vi "Tarea 17.vi"() -> ()   [LabVIEW 2019]
uses:
  Student Material/Student Material/Module 4/Exercises 17/CLD 17 Keypad_Typedef.ctl
panel:
  out "error out":errorcluster
  in  "error in (no error)":errorcluster
  out "Numeric":dbl
  in  "Keypad Cluster":T1
  out "String":string="0"
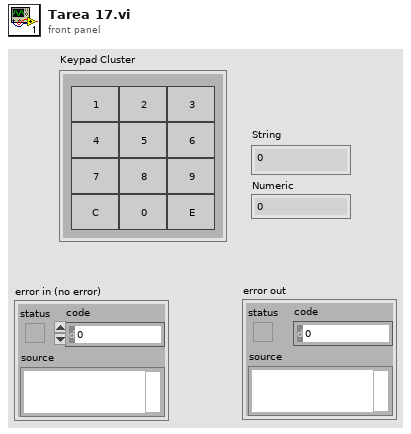
[diagram p1: front panel]
types:
  T1 = typedef "CLD 17 Keypad_Typedef.ctl" = cluster{"0":bool, "1":bool, "2":bool, "3":bool, "4":bool, "5":bool, "6":bool, "7":bool, "8":bool, "9":bool, "C":bool, "E":bool}
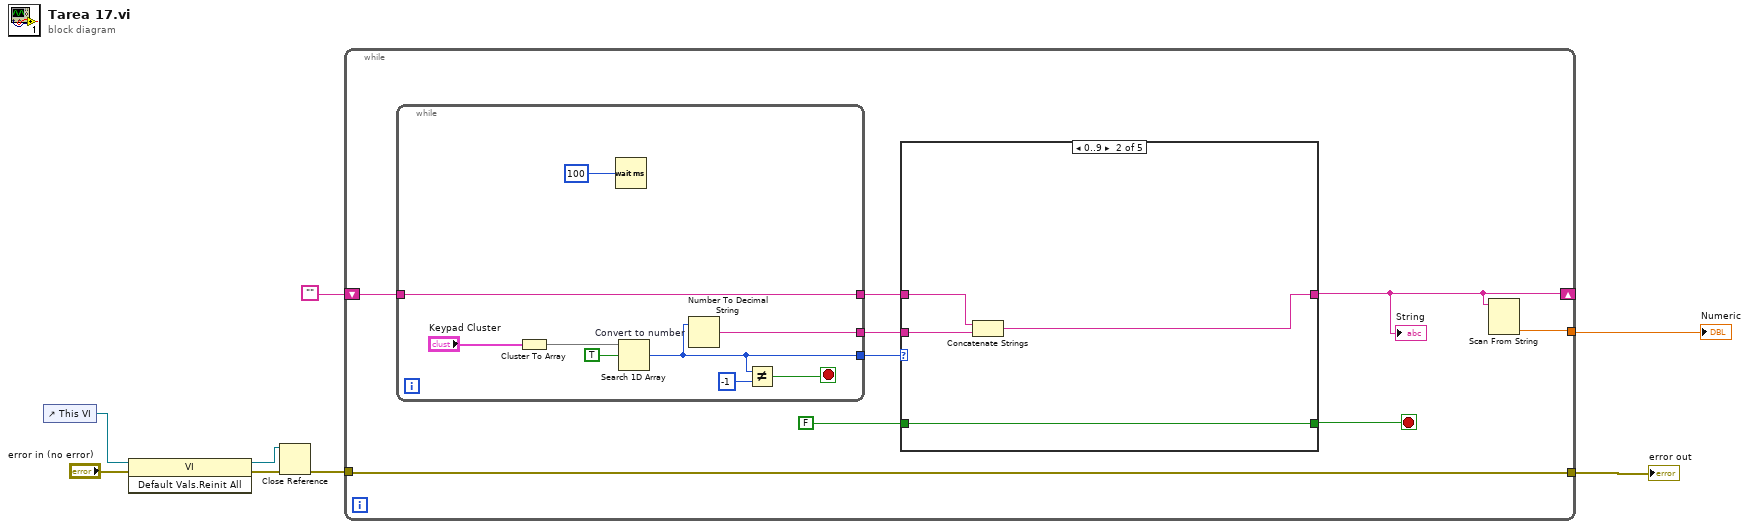
[diagram p0: block diagram]
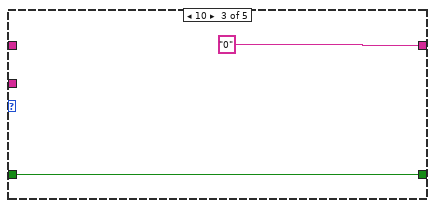
[diagram p3: hidden frame]
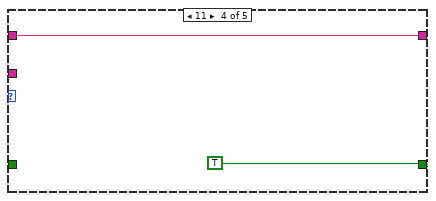
[diagram p4: hidden frame]
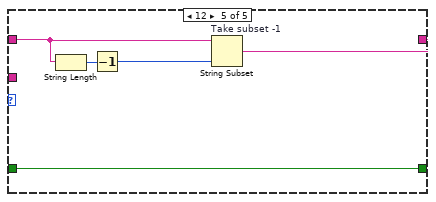
[diagram p5: hidden frame]
diagram:
  n1 = control-ref of="This VI"() -> (w7:refnum<vi>)
  n2 = invoke class="VI" method="Default Vals.Reinit All"(reference=w7, error in="error in (no error)") -> (reference out=w4:refnum<vi>, error out=w6:errorcluster)  [unwired: 1 in, 1 out]
  n3 = Close Reference(reference=w4, error in (no error)=w6) -> (error out=w5:errorcluster)
  n4 = while {
    shift-right: [w14] -> _
    shift-left: "" -> [w11]
    tunnel: w5 -> [w9]
    tunnel: [w17] -> w3
    tunnel: [w9] -> w1
    stop <- w13 stop-if-true
    n5 = while "Keypad Polling" {
      tunnel: [w34] -> w16
      tunnel: [w39] -> w15
      tunnel: [w38] -> w10
      tunnel: w11 -> [w38]
      stop <- w35 stop-if-true
      n6 = Cluster To Array(cluster="Keypad Cluster") -> (array=w36:bool[])
      n7 = Wait (ms)(milliseconds to wait=u32 100) -> ()  [unwired: 1 out]
      n8 = Search 1D Array(1D array=w36, element=TRUE) -> (index of element=w34:i32)  [unwired: 1 in]
      n9 = Number To Decimal String "Convert to number"(number=w34) -> (decimal integer string=w39:string)  [unwired: 1 in]
      n10 = Not Equal?(x=w34, y=-1) -> (x != y?=w35:bool)
    }
    n11 = case "Action Selector" shown="0..9" w16 {
      tunnel: w10 -> [w19 w23 _ w27 w29]
      tunnel: w15 -> [_ w22 _ _ _]
      tunnel: [w19 w21 "0" w27 w30] -> w14
      tunnel: [w18 w20 w25 TRUE w28] -> w13
      tunnel: FALSE ("Main Loop Exit?") -> [w18 w20 w25 _ w28]
      frame Default {
        # "Pass Sting"
      }
      frame 0..9 {
        n12 = Concatenate Strings(w23, w22) -> (w21:string)
      }
      frame 10 {
      }
      frame 11 {
      }
      frame 12 {
        n13 = String Length(string=w29) -> (length=w32:i32)
        n14 = Decrement(x=w32) -> (x-1=w31:i32)
        n15 = String Subset "Take subset -1"(string=w29, length (rest)=w31) -> (substring=w30:string)  [unwired: 1 in]
      }
    }
    "String" <- w14
    n16 = Scan From String(input string=w14) -> (output 1=w17:dbl)  [unwired: 4 in, 3 out]
  }
  "Numeric" <- w3
  "error out" <- w1
